vi "Create.vi"(8 "error in (no error)":errorcluster, 10 "WebView2 Control":refnum<k24>, 11 "Type":refnum<class "WebView2 Control.lvclass">) -> (0 "error out":errorcluster, 3 "WebView2 Control out":refnum<class "WebView2 Control.lvclass">)   [LabVIEW 2020, in "WebView2.lvlib" / "WebView2 Control.lvclass"]
uses:
  WebView2 Control.lvclass
  WebView2 Control.lvclass/WebView2 Control.ctl
  Source Changed Event Data.ctl
  Events.ctl
  Navigation Start Event Data.ctl
  C:/Users/Simon/Documents/GitHub/LV-WebView2/Source/Libs/Microsoft.Web.WebView2.Core.dll
  Libs/Microsoft.Web.WebView2.Core.dll
  Navigation Event Data.ctl
  <vilib>/Utility/sysdir.llb/System Directory Type.ctl
  Res.ctl
  C:/Users/Simon/Documents/GitHub/LV-WebView2/Source/Libs/Microsoft.Web.WebView2.WinForms.dll
  Libs/Microsoft.Web.WebView2.WinForms.dll
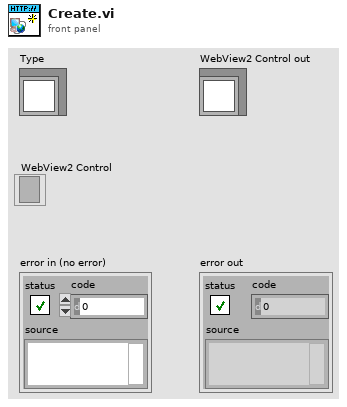
[diagram p1: front panel]
types:
  T1 = typedef "WebView2.lvlib/WebView2 Control.lvclass/Res.ctl" = cluster{"WebView2":refnum<k24>, "Webview2 Core":refnum<k24>, "event callback":refnum<k27>, "Environment":refnum<k24>}
  T2 = typedef "WebView2.lvlib/WebView2 Control.lvclass/Navigation Start Event Data.ctl" = cluster{"AdditionalAllowedFrameAncestors":string, "Cancel":bool, "IsRedirected":bool, "IsUserInitiated":bool, "NavigationId":u64, "NavigationKind":i32, "Uri":string, "Headers":cluster{"Key":string, "Value":string}[]}
  T3 = typedef "WebView2.lvlib/WebView2 Control.lvclass/Navigation Event Data.ctl" = cluster{"HttpStatusCode":i32, "IsSuccess":bool, "NavigationId":u64, "WebErrorStatus":i32}
  T4 = cluster{"Source":string, "WebMessageAsJson":string}
  T5 = typedef "WebView2.lvlib/WebView2 Control.lvclass/Events.ctl" = cluster{"Navigation Complete Event":refnum<user-event>, "Source Changed Event":refnum<user-event>, "Document Title Changed Event":refnum<user-event>, "Status Bar Text Changed":refnum<user-event>, "Web Message Received":refnum<user-event>, "Window Close Requested":refnum<user-event>, "DOM Loaded":refnum<user-event>, "Navigation Started Event":refnum<user-event>}
  T6 = typedef "System Directory Type.ctl" = i32
  T7 = typedef "WebView2.lvlib/WebView2 Control.lvclass/Source Changed Event Data.ctl" = cluster{"Source":string, "IsNewDocument":bool}
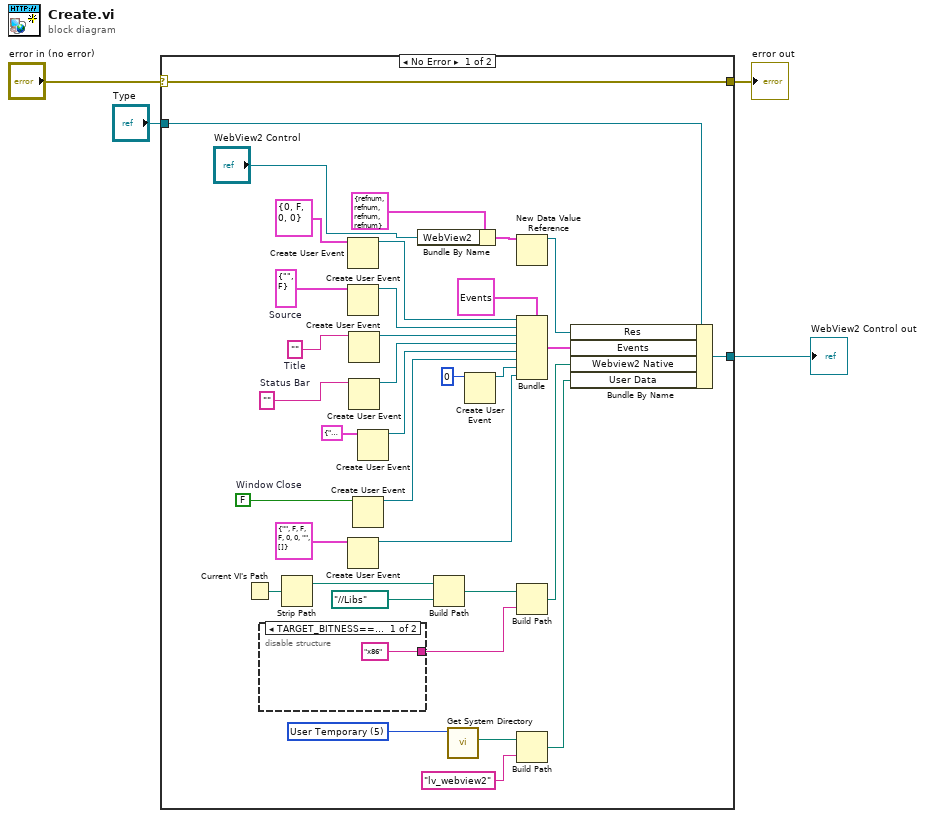
[diagram p0: block diagram]
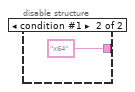
[diagram p2: hidden frame]
diagram:
  n1 = case shown="No Error" "error in (no error)" {
    selector: "error in (no error)" -> [w6 w43]
    tunnel: [w6 w43] -> w3
    tunnel: [w9 w42] -> w1
    tunnel: "Type" -> [w7 w42]
    frame No Error {
      w21 = T6 5 items=["User Home"=0, "User Desktop"=1, "User Documents"=2, "User Application Data"=3, "User Preferences"=4, "User Temporary"=5, "Public Documents"=6, "Public Application Data"=7, "Public Preferences"=8, "Public Cache"=13, "System Core Libraries"=9, "System Installed Libraries"=10, "Application Files"=11, "Boot Volume Root"=12] ("system directory type")
      w29 = FALSE  # Window Close
      w32 = ""  # Status Bar
      w38 = ""  # Title
      w39 = T7 {"Source"="", "IsNewDocument"=FALSE}  # Source
      n2 = Current VI's Path() -> (path=w26:path)
      n3 = disable-structure shown="TARGET_BITNESS==32, Default" {
        disable-tunnel: ["x86" "x64"] -> w23
        frame condition #0 (active) {
        }
        frame condition #1 {
        }
      }
      n4 = Strip Path(path=w26) -> (stripped path=w25:path)  [unwired: 1 out]
      n5 = Create User Event(user event datatype=T3 {"HttpStatusCode"=0, "IsSuccess"=FALSE, "NavigationId"=0, "WebErrorStatus"=0} ("output cluster")) -> (user event=w34:refnum<user-event>)  [unwired: 1 in, 1 out]
      n6 = Create User Event(user event datatype=w39) -> (user event=w33:refnum<user-event>)  [unwired: 1 in, 1 out]
      n7 = Create User Event(user event datatype=T2 {"AdditionalAllowedFrameAncestors"="", "Cancel"=FALSE, "IsRedirected"=FALSE, "IsUserInitiated"=FALSE, "NavigationId"=0, "NavigationKind"=0, "Uri"="", "Headers"=[]} ("Nav Started Event")) -> (user event=w13:refnum<user-event>)  [unwired: 1 in, 1 out]
      n8 = Create User Event(user event datatype=w38) -> (user event=w35:refnum<user-event>)  [unwired: 1 in, 1 out]
      n9 = Create User Event(user event datatype=w32) -> (user event=w31:refnum<user-event>)  [unwired: 1 in, 1 out]
      n10 = Create User Event(user event datatype=w29) -> (user event=w28:refnum<user-event>)  [unwired: 1 in, 1 out]
      n11 = Create User Event(user event datatype=T4 {"Source"="", "WebMessageAsJson"=""} ("output cluster")) -> (user event=w30:refnum<user-event>)  [unwired: 1 in, 1 out]
      n12 = Bundle By Name(cluster=T1 {"WebView2"=refnum, "Webview2 Core"=refnum, "event callback"=refnum, "Environment"=refnum} ("output cluster"), "WebView2"="WebView2 Control") -> (w8:T1)
      n13 = Build Path(base path=w25, name or relative path=path "../../Libs") -> (appended path=w22:path)
      n14 = call <vilib>:"Get System Directory.vi"("system directory type"=w21) -> ("system directory"=w20:path)  [unwired: 10 in]
      n15 = Create User Event(user event datatype=u64 0 ("NavigationId")) -> (user event=w16:refnum<user-event>)  [unwired: 1 in, 1 out]
      n16 = New Data Value Reference(data value=w8) -> (data value reference=w10:refnum<data-value>)  [unwired: 1 in, 1 out]
      n17 = Bundle(cluster=T5 {"Navigation Complete Event"=refnum, "Source Changed Event"=refnum, "Document Title Changed Event"=refnum, "Status Bar Text Changed"=refnum, "Web Message Received"=refnum, "Window Close Requested"=refnum, "DOM Loaded"=refnum, "Navigation Started Event"=refnum} ("Cluster"), "Navigation Complete Event"=w34, "Source Changed Event"=w33, "Document Title Changed Event"=w35, "Status Bar Text Changed"=w31, "Web Message Received"=w30, "Window Close Requested"=w28, "DOM Loaded"=w16, "Navigation Started Event"=w13) -> (w36:T5)
      n18 = Build Path(base path=w22, name or relative path=w23) -> (appended path=w18:path)
      n19 = Build Path(base path=w20, name or relative path="lv_webview2") -> (appended path=w17:path)
      n20 = Bundle By Name(cluster=w7, "Res"=w10, "Events"=w36, "Webview2 Native"=w18, "User Data"=w17) -> (w9:refnum<class "WebView2 Control.lvclass">)
    }
    frame Error {
    }
  }
  "error out" <- w3
  "WebView2 Control out" <- w1
